vi "Right To Feeder Station from Near Rocket.vi"   [LabVIEW 2018]
uses:
  Support Code/Path Data.ctl
  Framework/Robot Global Data.vi
types:
  T1 = typedef "Path Data.ctl" = cluster{"Maneuver":enum16{"MAX 90", "MAX 180", "Turn to Home", "Turn to Rocket", "Auto-Align", "Turn to ..."}, "Rotation Direction":enum16{"N/A", "Right", "Left"}}[]
  T2 = typedef "Command Status Info.ctl" = cluster{"Name":string, "Status":T3, "notifier out":T4}
  T3 = typedef "Completion Status.ctl" = enum16{"Successful", "Aborted", "Incomplete"}
  T4 = typedef "Completion Notifier.ctl" = refnum<notifier>
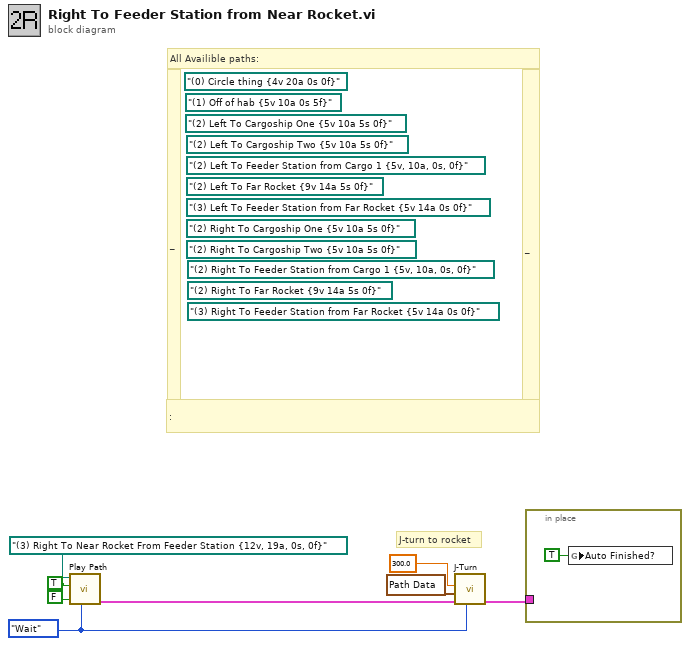
[diagram p0: block diagram]
diagram:
  w2 = enum16{"Start", "Wait"}."Wait" ("Synchronication")
  (unwired) path "(3) Right To Feeder Station from Far Rocket {5v 14a 0s 0f}"
  (unwired) path "(2) Right To Far Rocket {9v 14a 5s 0f}"
  (unwired) path "(2) Right To Feeder Station from Cargo 1 {5v, 10a, 0s, 0f}"
  (unwired) path "(2) Right To Cargoship Two {5v 10a 5s 0f}"
  (unwired) path "(2) Right To Cargoship One {5v 10a 5s 0f}"
  (unwired) path "(3) Left To Feeder Station from Far Rocket {5v 14a 0s 0f}"
  (unwired) path "(2) Left To Far Rocket {9v 14a 5s 0f}"
  (unwired) path "(2) Left To Feeder Station from Cargo 1 {5v, 10a, 0s, 0f}"
  (unwired) path "(2) Left To Cargoship Two {5v 10a 5s 0f}"
  (unwired) path "(2) Left To Cargoship One {5v 10a 5s 0f}"
  (unwired) path "(1) Off of hab {5v 10a 0s 5f}"
  (unwired) path "(0) Circle thing {4v 20a 0s 0f}"
  # "J-turn to rocket"
  # ":"
  # "_"
  # "_"
  # "All Availible paths:"
  n1 = call "Play Path.vi"("Synchronication"=w2, "Reverse (T) / Normal (F)"=FALSE, "Path Reversed"=TRUE, "Path"=path "(3) Right To Near Rocket From Feeder Station {12v, 19a, 0s, 0f}") -> ("Command Info Out"=w1:T2)  [unwired: 7 in]
  n2 = call "J-Turn.vi"("Synchronication"=w2, "Command Info In"=w1, "Path Data"=T1 [{"Maneuver"=enum."Turn to ...", "Rotation Direction"=enum."N/A"}, {"Maneuver"=enum."MAX 90", "Rotation Direction"=enum."N/A"}, {"Maneuver"=enum."MAX 90", "Rotation Direction"=enum."N/A"}], "Angle boi"=300.0) -> ("Command Info Out"=w6:T2)  [unwired: 7 in]
  n3 = in-place {
    in-place-border: w6 -> [_]
    n4 = global write "Robot Global Data.vi" "Auto Finished?"(TRUE ("Auto Finished?")) -> ()
  }
